vi "500 Internal Server Error.vi"(11 "LabVIEW Error Code":i32) -> (3 "Error":T1)   [LabVIEW 2016, in "ServerErrors.lvlib"]
uses:
  ServerErrors.lvlib
  Error Message--cluster.ctl
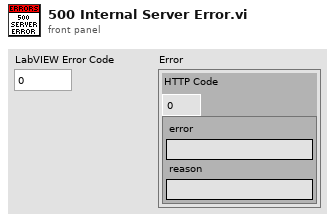
[diagram p1: front panel]
types:
  T1 = typedef "ServerErrors.lvlib/Error Message--cluster.ctl" = cluster{"HTTP Code":i32, "JSON Response":cluster{"error":string, "reason":string}}
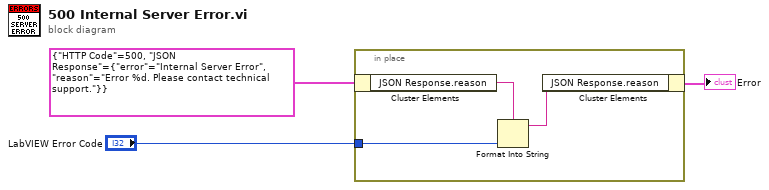
[diagram p0: block diagram]
diagram:
  n1 = in-place {
    in-place-border: "LabVIEW Error Code" -> [w5]
    n2 = in-place-cluster #1(T1 {"HTTP Code"=500, "JSON Response"={"error"="Internal Server Error", "reason"="Error %d. Please contact technical support."}} ("Error")) -> ("JSON Response.reason"=w6:string)
    n3 = Format Into String(format string=w6, w5) -> (resulting string=w4:string)  [unwired: 2 in, 1 out]
    n4 = in-place-cluster #1("JSON Response.reason"=w4) -> (→"Error":T1)
  }
